vi "PKCS1Padding.vi"(3 "error in (no error)":errorcluster, 4 "Message":string, 5 "Length":i32) -> (0 "error out":errorcluster, 1 "Hex (After Padding)":string)   [LabVIEW 2023]
uses:
  <vilib>/numeric/Random Number (Range) U64.vi
  <vilib>/numeric/sub_Random U32.vi
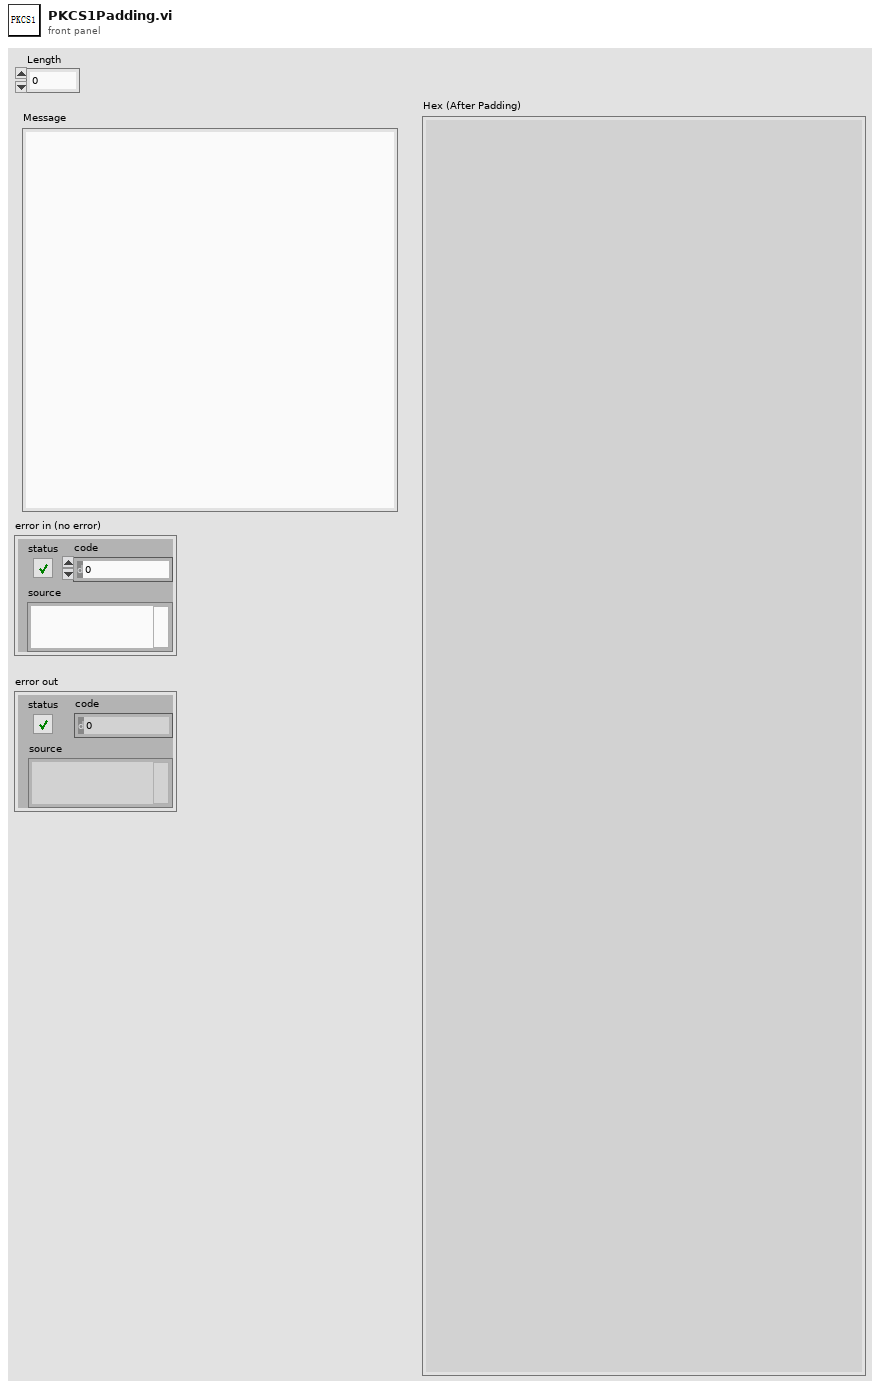
[diagram p1: front panel]
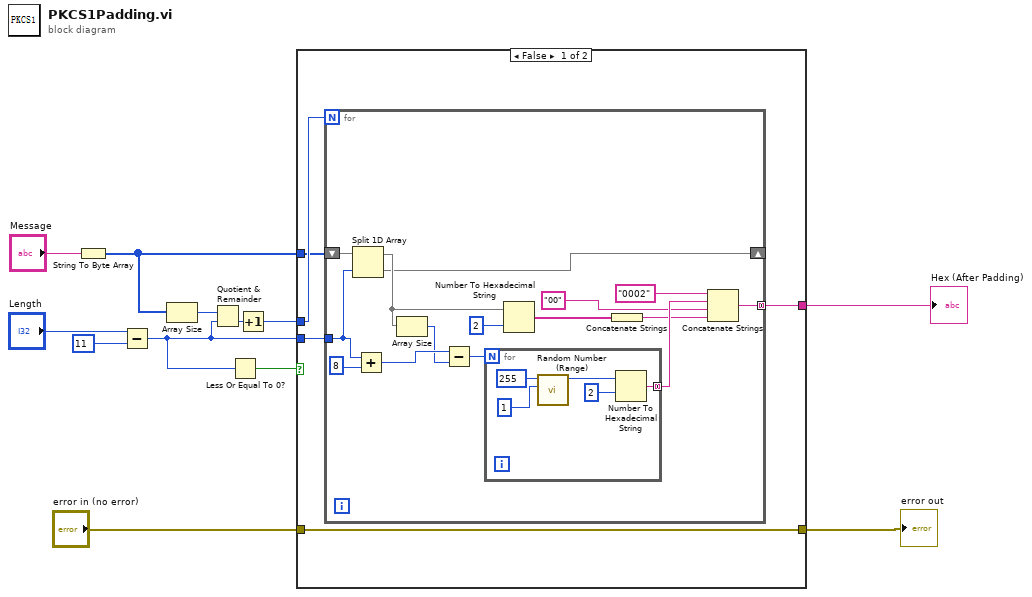
[diagram p0: block diagram]
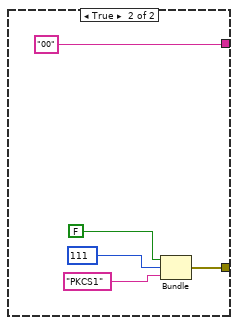
[diagram p2: hidden frame]
diagram:
  n1 = String To Byte Array(string="Message") -> (unsigned byte array=w5:u8[])
  n2 = Subtract(x="Length", y=11) -> (x-y=w6:i32)
  n3 = Array Size(array=w5) -> (size(s)=w7:i32)
  n4 = Quotient & Remainder(x=w7, y=w6) -> (floor(x/y)=w10:i32)  [unwired: 1 out]
  n5 = Less Or Equal To 0?(x=w6) -> (x <= 0?=w4:bool)
  n6 = Increment(x=w10) -> (x+1=w9:i32)
  n7 = case shown="False" w4 {
    tunnel: w9 -> [w17 _]
    tunnel: [w16 "00"] -> w1
    tunnel: w6 -> [w15 _]
    tunnel: w5 -> [w14 _]
    tunnel: "error in (no error)" -> [w13 _]
    tunnel: [w13 w38] -> w2
    frame False {
      n8 = for {
        N: w17 -> [_]
        tunnel: w15 -> [w26]
        tunnel: [w29] -> w16 mode=concatenating
        shift-right: [w21] -> _
        shift-left: w14 -> [w28]
        n9 = Split 1D Array(array=w28, index=w26) -> (first subarray=w22:u8[], second subarray=w21:u8[])
        n10 = Add(x=w26, y=8) -> (x+y=w20:i32)
        n11 = Array Size(array=w22) -> (size(s)=w19:i32)
        n12 = Subtract(x=w20, y=w19) -> (x-y=w24:i32)
        n13 = for {
          N: w24 -> [_]
          tunnel: [w33] -> w31 mode=concatenating
          n14 = call-poly <vilib>:"Random Number (Range).vi"("lower bound (0)"=u64 1, "upper bound (100)"=u64 255) -> ("number"=w35:u64)  [unwired: 9 in]
          n15 = Number To Hexadecimal String(1:2, 2:w35) -> (0:w33:string)
        }
        n16 = Number To Hexadecimal String(1:2, 2:w22) -> (0:w27:string[])
        n17 = Concatenate Strings(w27) -> (w23:string)
        n18 = Concatenate Strings("0002", w31, "00", w23) -> (w29:string)
      }
    }
    frame True {
      n19 = Bundle(FALSE, 111, "PKCS1") -> (w38:errorcluster)  [unwired: 1 in]
    }
  }
  "Hex (After Padding)" <- w1
  "error out" <- w2
